vi "svl_Peak Level with IC_octave.vi"(2 "init/cont (init:F)":bool, 3 "initial peak level":dbl format="%.2f", 4 "scaled signal [EU]":dbl[](array[numeric]) format="%.2f") -> (0 "final peak level":dbl format="%.2f", 1 "peak level":dbl format="%.2f")   [LabVIEW 2017]
doc: "Detects the peak level based on the input signal and the initial peak level.\nThe initial peak level and the final peak level parameters keep track of the internal state of the peak detection process to ensure continuous operation if continuous mode is used."
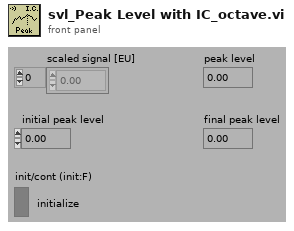
[diagram p1: front panel]
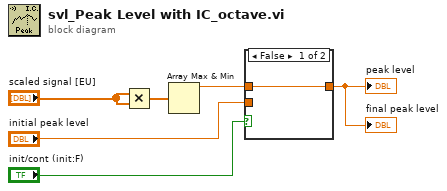
[diagram p0: block diagram]
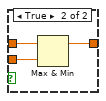
[diagram p2: hidden frame]
diagram:
  n1 = Multiply(x="scaled signal [EU]", y="scaled signal [EU]") -> (x*y=w5:dbl[])
  n2 = Array Max & Min(array=w5) -> (max value=w1:dbl)  [unwired: 3 out]
  n3 = case shown="False" "init/cont (init:F)" {
    tunnel: w1 -> [w7 w10]
    tunnel: [w7 w8] -> w2
    tunnel: "initial peak level" -> [_ w9]
    frame False {
    }
    frame True {
      n4 = Max & Min(x=w10, y=w9) -> (max(x,y)=w8:dbl)  [unwired: 1 out]
    }
  }
  "peak level" <- w2
  "final peak level" <- w2
